vi "Tempo de processamento.vi"() -> ()   [LabVIEW 2018]
panel:
  out "Time":dbl format="%#_2f"
  out "# of iterations":dbl
  out "Current number":dbl
  in  "Number to match":dbl
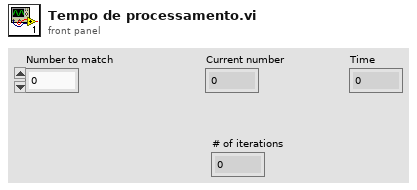
[diagram p1: front panel]
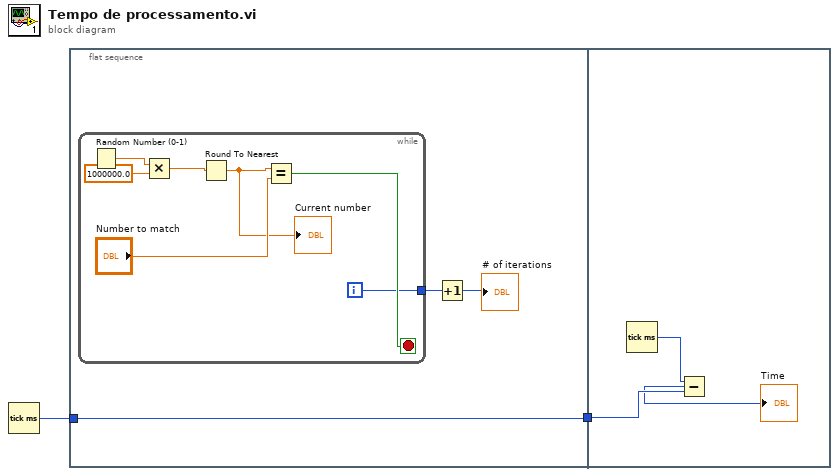
[diagram p0: block diagram]
diagram:
  n1 = Tick Count (ms)() -> (millisecond timer value=w2:u32)
  n2 = flat-sequence {
    tunnel: w2 -> [w3]
    tunnel: [w3] -> w1
    tunnel: w1 -> [w14]
    frame #0 {
      n3 = while {
        tunnel: [w6] -> w5
        i -> [w6]
        stop <- w7 stop-if-true
        n4 = Random Number (0-1)() -> (number: 0 to 1=w12:dbl)
        n5 = Multiply(x=w12, y=1000000.0) -> (x*y=w10:dbl)
        n6 = Round To Nearest(number=w10) -> (nearest integer value=w8:dbl)
        "Current number" <- w8
        n7 = Equal?(x=w8, y="Number to match") -> (x = y?=w7:bool)
      }
      n8 = Increment(x=w5) -> (x+1=→"# of iterations":i32)
    }
    frame #1 {
      n9 = Tick Count (ms)() -> (millisecond timer value=w15:u32)
      n10 = Subtract(x=w15, y=w14) -> (x-y=→"Time":u32)
    }
  }
